vi "Get Messages.vi"(7 "Visibility timeout (30 seconds)":u32=30, 8 "error in (no error)":errorcluster, 9 "Number of messages (1)":u32=1, 10 "Queue":string, 11 "Azure Session in":refnum<class "Session.lvclass">) -> (0 "error out":errorcluster, 2 "Messages":T1[](array[typedef]), 3 "Azure Session out":refnum<class "Session.lvclass">)   [LabVIEW 2015, in "NI_Azure_Queue.lvlib"]
doc: "Retrieves a message from the queue and makes it invisible to other consumers."
uses:
  NI_Azure_Queue.lvlib
  Core/Session/Session.lvclass
  Message.ctl
  Core/Name Value Pair.ctl
  Core/Session/Session.lvclass/Session.ctl
  Core/Session/Write HTTP Verb.vi
  Core/Session/Write URL Suffix.vi
  Core/Session/Write Request Parameters.vi
  Core/NI_Azure_Core.lvlib
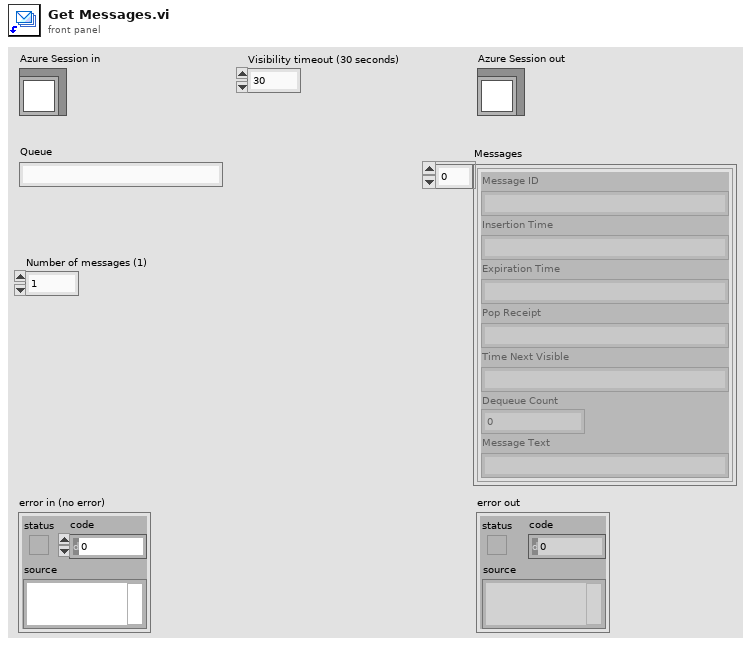
[diagram p1: front panel]
types:
  T1 = typedef "NI_Azure_Queue.lvlib/Message.ctl" = cluster{"Message ID":string, "Insertion Time":string, "Expiration Time":string, "Pop Receipt":string, "Time Next Visible":string, "Dequeue Count":i32, "Message Text":string}
  T2 = typedef "NI_Azure_Core.lvlib/Name Value Pair.ctl" = cluster{"name":string, "value":string}
  T3 = typedef "NI_Azure_Core.lvlib/Response.ctl" = cluster{"Headers":string, "Body":string}
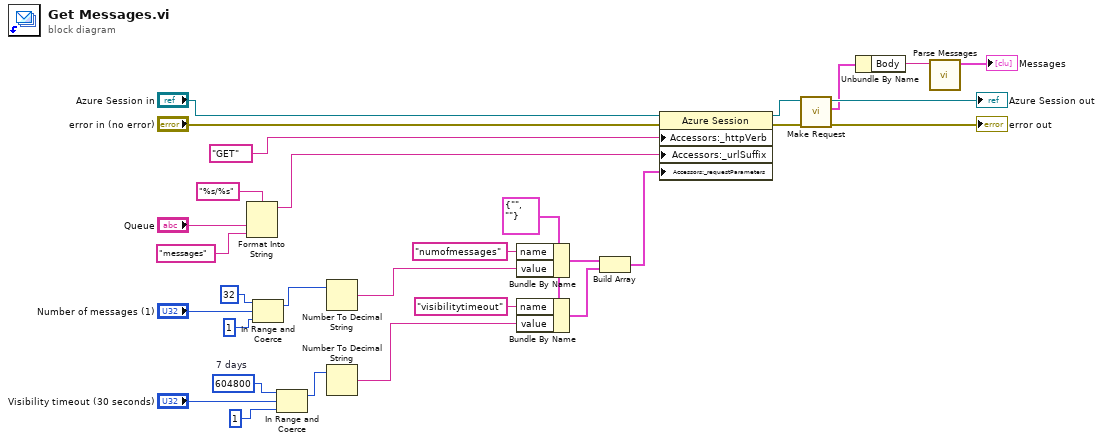
[diagram p0: block diagram]
diagram:
  w9 = T2 {"name"="", "value"=""} ("Name Value Pair")
  w11 = u32 604800  # 7 days
  n1 = Format Into String(format string="%s/%s", "Queue", "messages") -> (resulting string=w21:string)  [unwired: 2 in, 1 out]
  n2 = In Range and Coerce(upper limit=u32 32, x="Number of messages (1)", lower limit=u32 1) -> (coerced(x)=w4:u32)  [unwired: 1 out]
  n3 = In Range and Coerce(upper limit=w11, x="Visibility timeout (30 seconds)", lower limit=u32 1) -> (coerced(x)=w2:u32)  [unwired: 1 out]
  n4 = Number To Decimal String(number=w4) -> (decimal integer string=w3:string)  [unwired: 1 in]
  n5 = Number To Decimal String(number=w2) -> (decimal integer string=w1:string)  [unwired: 1 in]
  n6 = Bundle By Name(cluster=w9, "name"="numofmessages", "value"=w3) -> (w7:T2)
  n7 = Bundle By Name(cluster=w9, "name"="visibilitytimeout", "value"=w1) -> (w6:T2)
  n8 = Build Array(w7, w6) -> (w5:T2[])
  n9 = property class="Azure Session"(reference="Azure Session in", error in="error in (no error)", "Accessors:_httpVerb"="GET" ("HTTP-Verb"), "Accessors:_urlSuffix"=w21, "Accessors:_requestParameters"=w5) -> (reference out=w22:refnum<class "Session.lvclass">, error out=w24:errorcluster)
  n10 = call "Make Request.vi"("error in (no error)"=w24, "Session in"=w22) -> ("error out"=→"error out":errorcluster, "Response"=w25:T3, "Session out"=→"Azure Session out":refnum<class "Session.lvclass">)  [unwired: 7 in]
  n11 = Unbundle By Name(w25) -> ("Body"=w18:string)
  n12 = call "Parse Messages.vi"("Body"=w18) -> ("Messages"=→"Messages":T1[])  [unwired: 10 in]
